vi "Find_Valid_Destination.vi"(8 "error in (no error)":errorcluster, 10 "Destinations in":refnum<class "AB_Destination.lvclass">[](array[class]), 11 "AB_Source in":refnum<class "AB_Source.lvclass">) -> (0 "error out":errorcluster, 1 "destinationIndex":i32, 2 "Destinations out":refnum<class "AB_Destination.lvclass">[](array[class]), 3 "AB_Source out":refnum<class "AB_Source.lvclass">, 5 "createdDestination?":bool)   [LabVIEW 2020, in "AB_Source.lvclass"]
uses:
  <vilib>/AppBuilder/AB_Classes/Source/AB_Source.lvclass
  <vilib>/AppBuilder/AB_Classes/Destination/AB_Destination.lvclass
  <vilib>/AppBuilder/AB_Classes/Source/AB_Source.lvclass/AB_Source.ctl
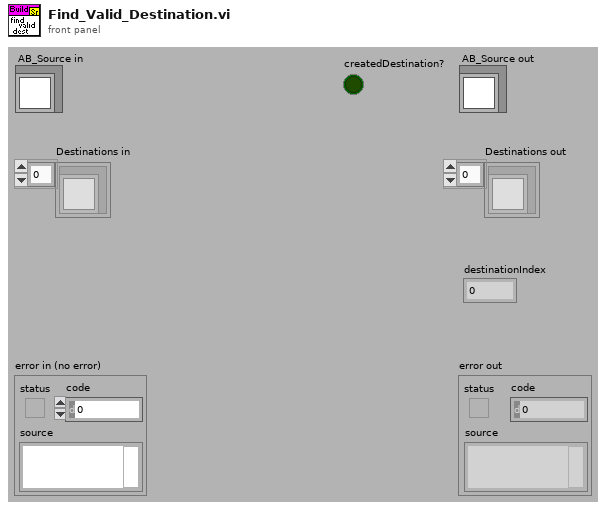
[diagram p1: front panel]
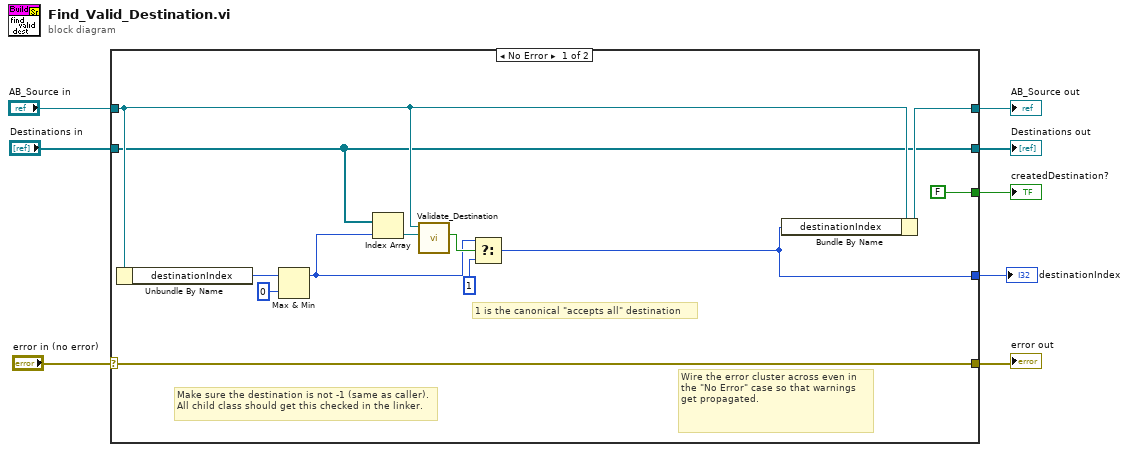
[diagram p0: block diagram]
diagram:
  n1 = case shown="No Error" "error in (no error)" {
    selector: "error in (no error)" -> [w20 w23]
    tunnel: [w20 w23] -> w7
    tunnel: [w18 w22] -> w5
    tunnel: "AB_Source in" -> [w15 w22]
    tunnel: [w14 w21] -> w4
    tunnel: "Destinations in" -> [w14 w21]
    tunnel: [FALSE _] -> w2
    tunnel: [w9 _] -> w1
    frame No Error {
      # "1 is the canonical \"accepts all\" destination"
      # "Make sure the destination is not -1 (same as caller). All child class should get this checked in the linker."
      # "Wire the error cluster across even in the \"No Error\" case so that warnings get propagated."
      n2 = Unbundle By Name(w15) -> ("destinationIndex"=w17:i32)
      n3 = Max & Min(x=w17, y=0) -> (max(x,y)=w11:i32)  [unwired: 1 out]
      n4 = Index Array(array=w14, index=w11) -> (element=w13:refnum<class "AB_Destination.lvclass">)
      n5 = call <vilib>:"Validate_Destination.vi"("Destination"=w13, "AB_Source in"=w15) -> ("Valid"=w12:bool)  [unwired: 7 in, 2 out]
      n6 = Select(t=w11, s=w12, f=1) -> (s? t:f=w9:i32)
      n7 = Bundle By Name(cluster=w15, "destinationIndex"=w9) -> (w18:refnum<class "AB_Source.lvclass">)
    }
    frame Error {
    }
  }
  "error out" <- w7
  "AB_Source out" <- w5
  "Destinations out" <- w4
  "createdDestination?" <- w2
  "destinationIndex" <- w1
